vi "Save Settings.vi"(8 "error in (no error)":errorcluster, 11 "GlobalData":T1) -> (0 "error out":errorcluster)   [LabVIEW 2024]
doc: "This VI used to save data to config file"
uses:
  controls/GlobalData.ctl
  <vilib>/Utility/config.llb/Write Key (String).vi
  <vilib>/Utility/config.llb/NI_LVConfig.lvlib
panel:
  out "success":bool
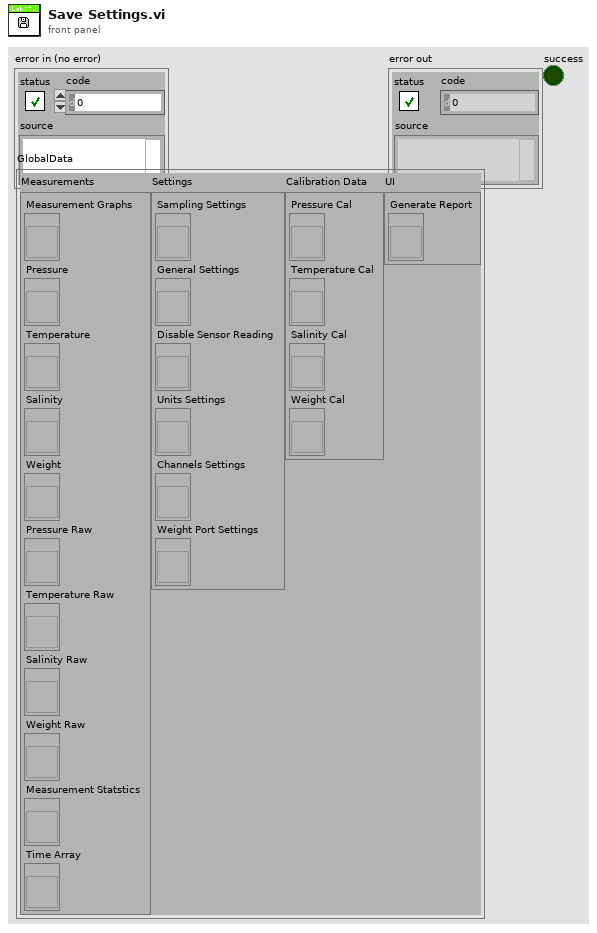
[diagram p1: front panel]
types:
  T1 = typedef "GlobalData.ctl" = cluster{"Measurements":cluster{"Measurement Graphs":refnum<vi>, "Pressure":refnum<vi>, "Temperature":refnum<vi>, "Salinity":refnum<vi>, "Weight":refnum<vi>, "Pressure Raw":refnum<vi>, "Temperature Raw":refnum<vi>, "Salinity Raw":refnum<vi>, "Weight Raw":refnum<vi>, "Measurement Statstics":refnum<vi>, "Time Array":refnum<vi>}, "Settings":cluster{"Sampling Settings":refnum<vi>, "General Settings":refnum<vi>, "Disable Sensor Reading":refnum<vi>, "Units Settings":refnum<vi>, "Channels Settings":refnum<vi>, "Weight Port Settings":refnum<vi>}, "Calibration Data":cluster{"Pressure Cal":refnum<vi>, "Temperature Cal":refnum<vi>, "Salinity Cal":refnum<vi>, "Weight Cal":refnum<vi>}, "UI":cluster{"Generate Report":refnum<vi>}}
  T2 = cluster{"Pressure":cluster{"Physical Channel":tag, "Min Voltage":dbl, "Max Voltage ":dbl, "Terminal Configuration":i32}, "Temperature":cluster{"Physical Channel":tag, "Min Current (mA)":dbl, "Max Current (mA)":dbl, "Terminal Configuration":i32}, "Sallinity":cluster{"Physical Channel":tag, "Min Current (mA)":dbl, "Max Current (mA)":dbl, "Terminal Configuration":i32}}
  T3 = typedef "Serial - Settings.ctl" = cluster{"baud rate":u32, "data bits":u16, "parity":enum16{"None", "Odd", "Even", "Mark", "Space"}, "stop bits":u16, "flow control":u16}
  T4 = cluster{"Port Name":refnum<visa-resource-name>, "Port Settings":T3}
  T5 = typedef "Units.ctl" = cluster{"Pressure":enum16{"PSI", "Bar", "atm", "Pa"}, "Temperature":enum16{"C", "K", "F"}, "Salinity":enum16{"ppm", "ppt", "PSU"}, "Weight":enum16{"Kg", "g", "oz", "ib"}}
  T6 = cluster{"Measurement Statstics":bool, "Logging Type":enum16{"Disable Log", "TDMS", "CSV"}}
  T7 = cluster{"Reading Time (ms)":u64, "Graph Time ":u16}
  T8 = typedef "NI_LVConfig.lvlib/Config Data RefNum.ctl" = refnum<k1>
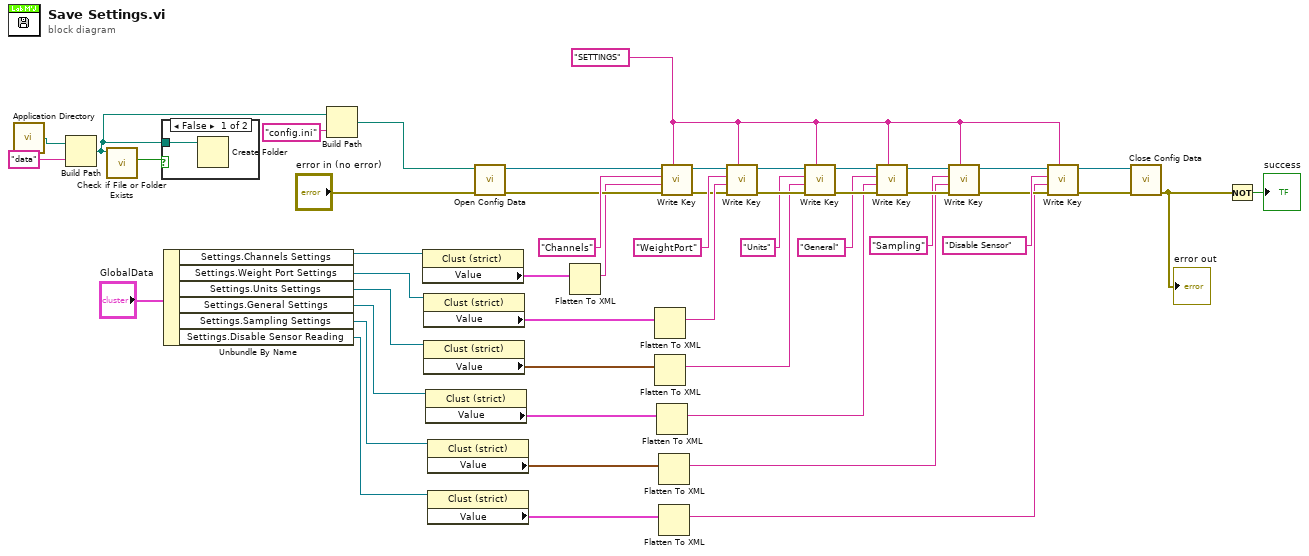
[diagram p0: block diagram]
diagram:
  w14 = "SETTINGS" ("section")
  n1 = call <vilib>:"Application Directory.vi"() -> ("Application Directory"=w5:path)
  n2 = Build Path(base path=w5, name or relative path="data") -> (appended path=w3:path)
  n3 = call <vilib>:"Check if File or Folder Exists.vi"("path"=w3) -> ("file or folder exists?"=w4:bool)  [unwired: 8 in, 2 out]
  n4 = case shown="False" w4 {
    tunnel: w3 -> [w50 _]
    frame False {
      n5 = Create Folder(path (use dialog)=w50) -> ()  [unwired: 2 in, 3 out]
    }
    frame True {
    }
  }
  n6 = Unbundle By Name("GlobalData") -> ("Settings.Channels Settings"=w31:refnum<vi>, "Settings.Weight Port Settings"=w30:refnum<vi>, "Settings.Units Settings"=w21:refnum<vi>, "Settings.General Settings"=w22:refnum<vi>, "Settings.Sampling Settings"=w23:refnum<vi>, "Settings.Disable Sensor Reading"=w10:refnum<vi>)
  n7 = Build Path(base path=w3, name or relative path="config.ini") -> (appended path=w2:path)
  n8 = property class="Clust (strict)"(reference=w31) -> ("Value"=w43:T2)  [unwired: 1 in, 2 out]
  n9 = property class="Clust (strict)"(reference=w30) -> ("Value"=w39:T4)  [unwired: 1 in, 2 out]
  n10 = property class="Clust (strict)"(reference=w21) -> ("Value"=w26:T5)  [unwired: 1 in, 2 out]
  n11 = property class="Clust (strict)"(reference=w22) -> ("Value"=w25:T6)  [unwired: 1 in, 2 out]
  n12 = property class="Clust (strict)"(reference=w23) -> ("Value"=w24:T7)  [unwired: 1 in, 2 out]
  n13 = property class="Clust (strict)"(reference=w10) -> ("Value"=w11:cluster{"Daq":bool, "RS232":bool})  [unwired: 1 in, 2 out]
  n14 = call <vilib>:"Open Config Data.vi"("error in (no error)"="error in (no error)", "configuration file path"=w2) -> ("error out"=w47:errorcluster, "refnum"=w49:T8)  [unwired: 7 in, 1 out]
  n15 = Flatten To XML(6:w43) -> (2:w42:string)
  n16 = Flatten To XML(6:w39) -> (2:w38:string)
  n17 = Flatten To XML(6:w26) -> (2:w20:string)
  n18 = Flatten To XML(6:w25) -> (2:w19:string)
  n19 = Flatten To XML(6:w24) -> (2:w18:string)
  n20 = Flatten To XML(6:w11) -> (2:w9:string)
  n21 = call-poly <vilib>:"Write Key.vi"("section"=w14, "error in (no error)"=w47, "value"=w42, "key"="Channels", "refnum"=w49) -> ("error out"=w1:errorcluster, "refnum out"=w40:T8)  [unwired: 4 in, 1 out]
  n22 = call-poly <vilib>:"Write Key.vi"("section"=w14, "error in (no error)"=w1, "value"=w38, "key"="WeightPort", "refnum"=w40) -> ("error out"=w36:errorcluster, "refnum out"=w37:T8)  [unwired: 4 in, 1 out]
  n23 = call-poly <vilib>:"Write Key.vi"("section"=w14, "error in (no error)"=w36, "value"=w20, "key"="Units", "refnum"=w37) -> ("error out"=w34:errorcluster, "refnum out"=w35:T8)  [unwired: 4 in, 1 out]
  n24 = call-poly <vilib>:"Write Key.vi"("section"=w14, "error in (no error)"=w34, "value"=w19, "key"="General", "refnum"=w35) -> ("error out"=w32:errorcluster, "refnum out"=w33:T8)  [unwired: 4 in, 1 out]
  n25 = call-poly <vilib>:"Write Key.vi"("section"=w14, "error in (no error)"=w32, "value"=w18, "key"="Sampling", "refnum"=w33) -> ("error out"=w16:errorcluster, "refnum out"=w15:T8)  [unwired: 4 in, 1 out]
  n26 = call-poly <vilib>:"Write Key.vi"("section"=w14, "error in (no error)"=w16, "value"=w9, "key"="Disable Sensor", "refnum"=w15) -> ("error out"=w12:errorcluster, "refnum out"=w13:T8)  [unwired: 4 in, 1 out]
  n27 = call <vilib>:"Close Config Data.vi"("error in (no error)"=w12, "refnum"=w13) -> ("error out"=w45:errorcluster)  [unwired: 8 in, 1 out]
  "error out" <- w45
  n28 = Not(x=w45) -> (.not. x?=→"success":bool)
